vi "svx_Pass Reset to Next Iteration.vi"(9 "trigger":bool, 10 "reset?(F)":bool) -> (2 "reset out":bool)   [LabVIEW 2017]
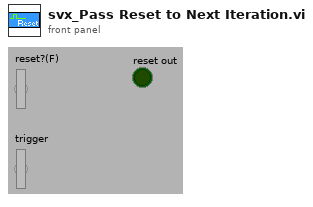
[diagram p1: front panel]
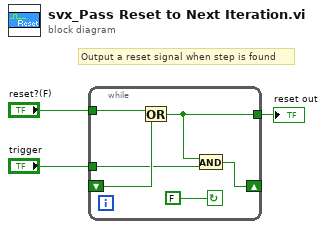
[diagram p0: block diagram]
diagram:
  # "Output a reset signal when step is found"
  n1 = while {
    tunnel: "reset?(F)" -> [w8]
    tunnel: "trigger" -> [w4]
    shift-right: [w5] -> _
    shift-left: _ -> [w7]
    tunnel: [w6] -> w2
    stop <- FALSE continue-if-true
    n2 = Or(x=w8, y=w7) -> (x .or. y?=w6:bool)
    n3 = And(x=w6, y=w4) -> (x .and. y?=w5:bool)
  }
  "reset out" <- w2
